vi "Setup.vi"(1 "error in":errorcluster caption="错误输入（无错误）") -> (2 "参数输出":T2={"帧ID1"=0, "等待延时"=0, "间隔延时"=0, "总时间"=0, "总次数"=0, "发送数据1"="", "接收数据1"="", "发送数据2"="", "接收数据2"="", "CAN盒类型"=3, "帧ID2"=0, "同步启动个数"=8, "模式"=enum."整体", "Baud"=12} {"Baud" items=["250k bps"=10, "10k bps"=2, "5k bps"=1, "50k bps"=5, "40k bps"=4, "20k bps"=3, "80k bps"=6, "100k bps"=7, "125k bps"=8, "200k bps"=9, "400k bps"=11, "500k bps"=12, "666k bps"=13, "800k bps"=14, "1000k bps"=15]; "帧ID2" format="%.0x"; "CAN盒类型" items=["PCI-CAN200"=7, "USB-CAN"=2, "USB-CAN200"=3]; "帧ID1" format="%.0x"}, 3 "Modify?":bool, 4 "原始参数":T2 {"CAN盒类型" items=["PCI-CAN200"=7, "USB-CAN"=2, "USB-CAN200"=3]}, 5 "error out":errorcluster caption="错误输出")   [LabVIEW 2013]
uses:
  USBCAN/DevType.ctl
panel:
  in  "输出簇":T3
  in  "Cancel":bool
  in  "Save":bool
  in  "测试参数":T2={"帧ID1"=0, "等待延时"=0, "间隔延时"=10, "总时间"=0, "总次数"=0, "发送数据1"="", "接收数据1"="", "发送数据2"="", "接收数据2"="", "CAN盒类型"=3, "帧ID2"=0, "同步启动个数"=8, "模式"=enum."整体", "Baud"=12} {"Baud" items=["250k bps"=10, "10k bps"=2, "5k bps"=1, "50k bps"=5, "40k bps"=4, "20k bps"=3, "80k bps"=6, "100k bps"=7, "125k bps"=8, "200k bps"=9, "400k bps"=11, "500k bps"=12, "666k bps"=13, "800k bps"=14, "1000k bps"=15]; "帧ID2" max=4096 step=1 format="%.0x"; "同步启动个数" min=1 max=8 step=1; "CAN盒类型" items=["PCI-CAN200"=7, "USB-CAN"=2, "USB-CAN200"=3]; "间隔延时" min=1 max=50 step=1; "帧ID1" max=4096 step=1 format="%.0x"}
  # "ms"
  # "ms"
  # "s"
  # "ms"
  # "ms"
  # "s"
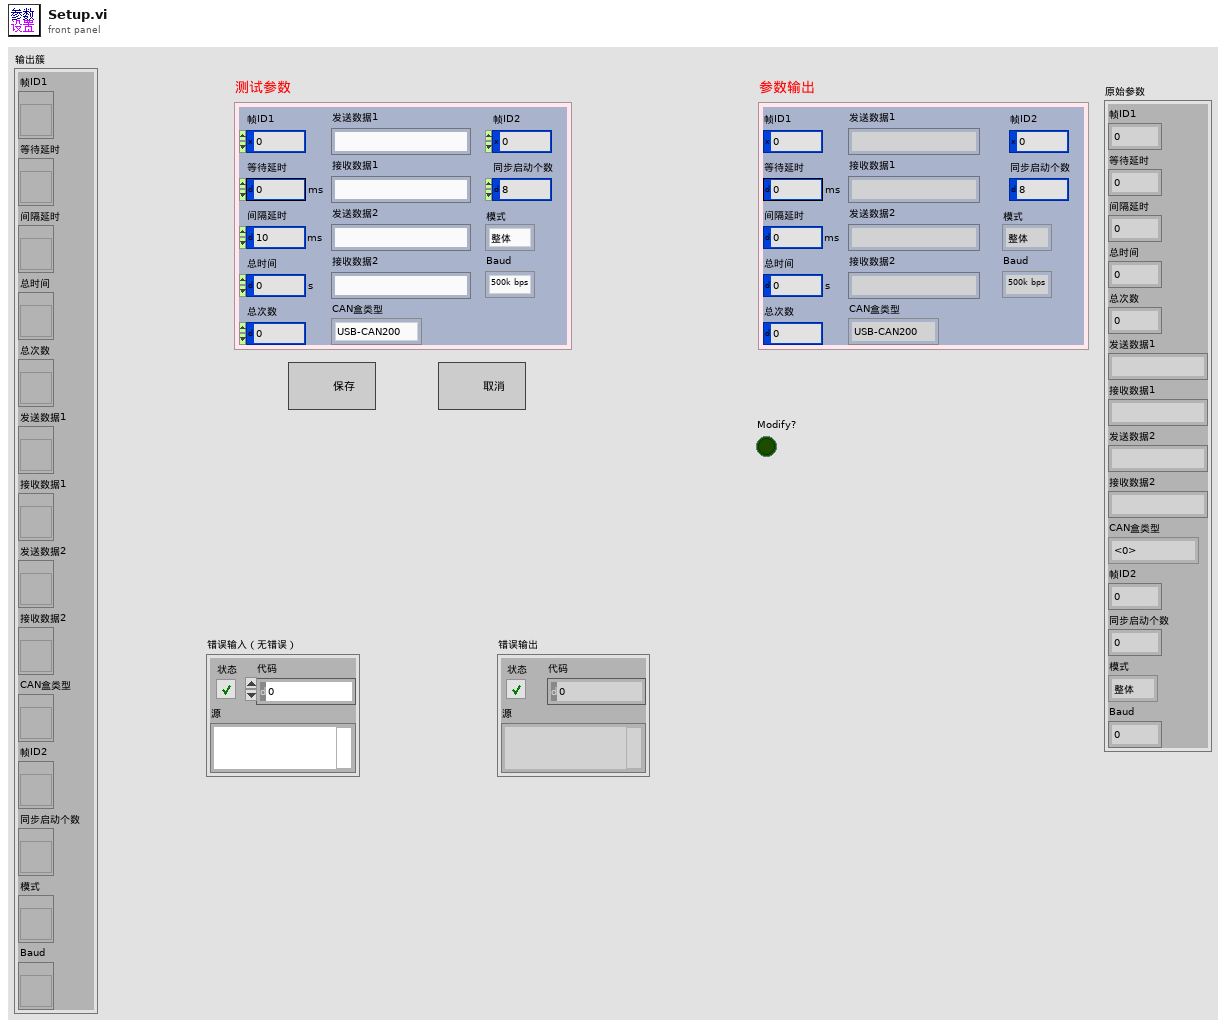
[diagram p1: front panel]
types:
  T1 = typedef "DevType.ctl" = u16
  T2 = cluster{"帧ID1":u32, "等待延时":u32, "间隔延时":u32, "总时间":u32, "总次数":u32, "发送数据1":string, "接收数据1":string, "发送数据2":string, "接收数据2":string, "CAN盒类型":T1, "帧ID2":u32, "同步启动个数":u8, "模式":enum16{"整体", "单个"}, "Baud":u8}
  T3 = cluster{"帧ID1":refnum<vi>, "等待延时":refnum<vi>, "间隔延时":refnum<vi>, "总时间":refnum<vi>, "总次数":refnum<vi>, "发送数据1":refnum<vi>, "接收数据1":refnum<vi>, "发送数据2":refnum<vi>, "接收数据2":refnum<vi>, "CAN盒类型":refnum<vi>, "帧ID2":refnum<vi>, "同步启动个数":refnum<vi>, "模式":refnum<vi>, "Baud":refnum<vi>}
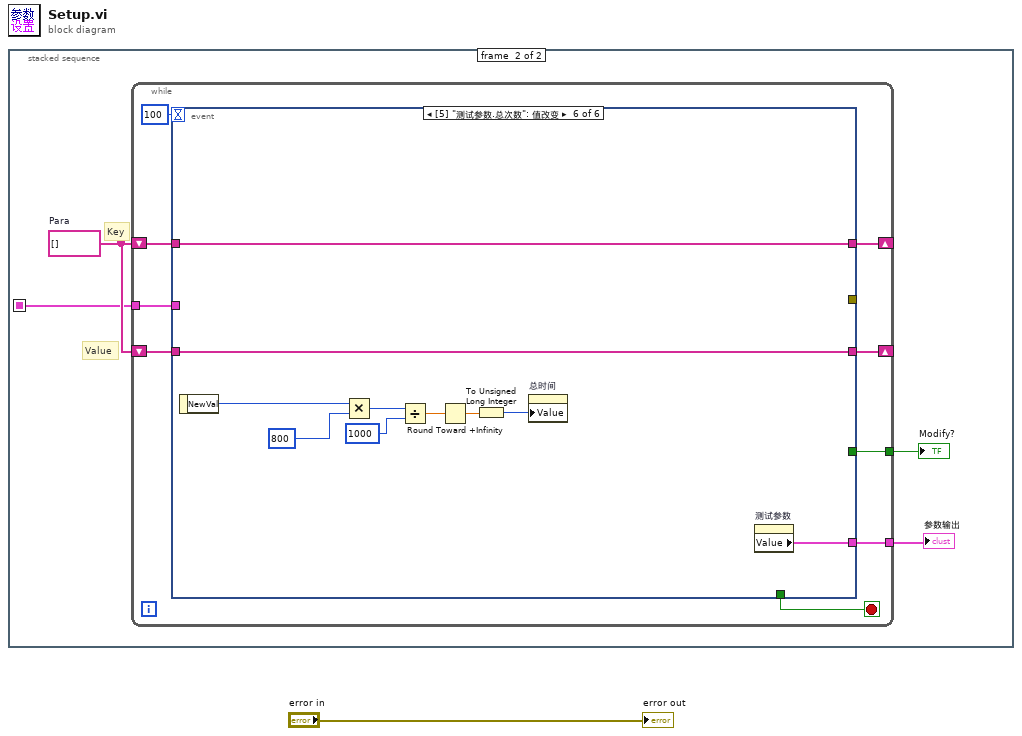
[diagram p0: block diagram]
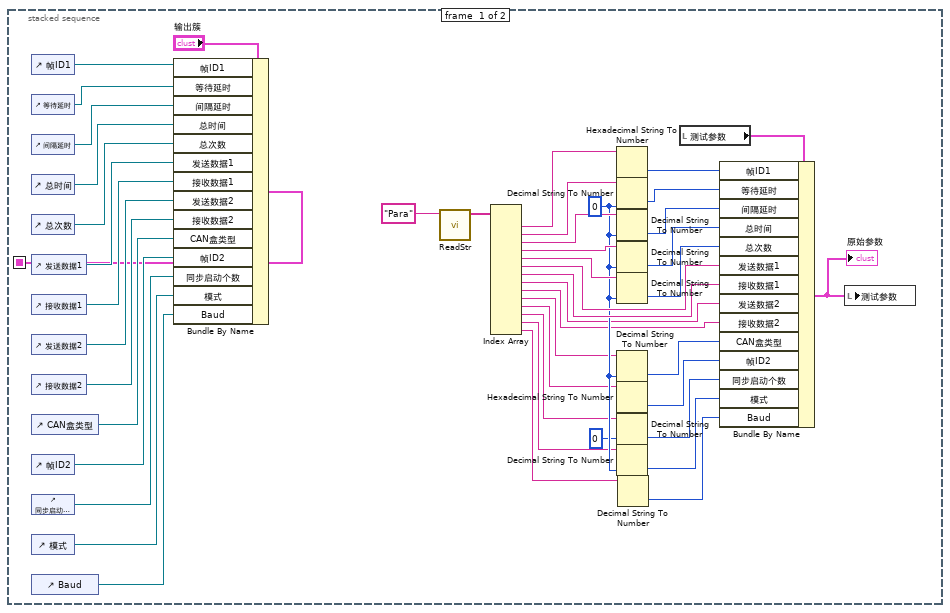
[diagram p2: hidden frame]
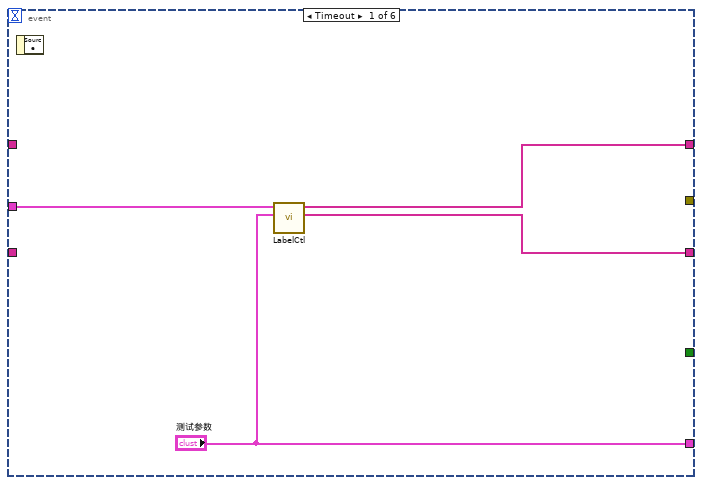
[diagram p3: hidden frame]
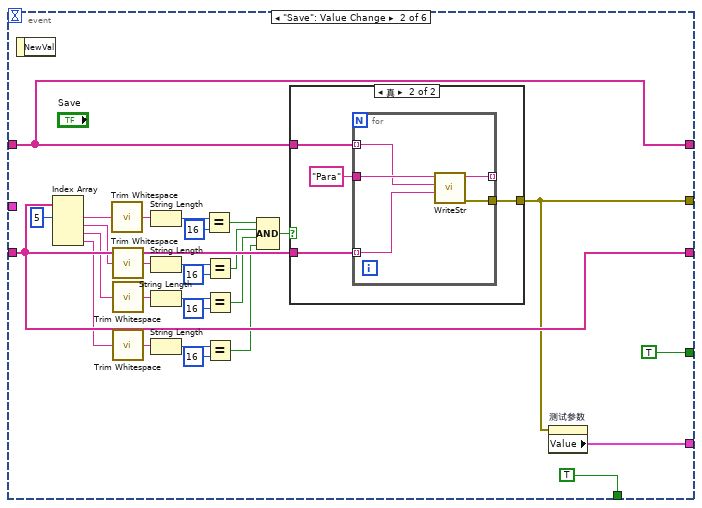
[diagram p4: hidden frame]
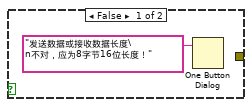
[diagram p5: hidden frame]
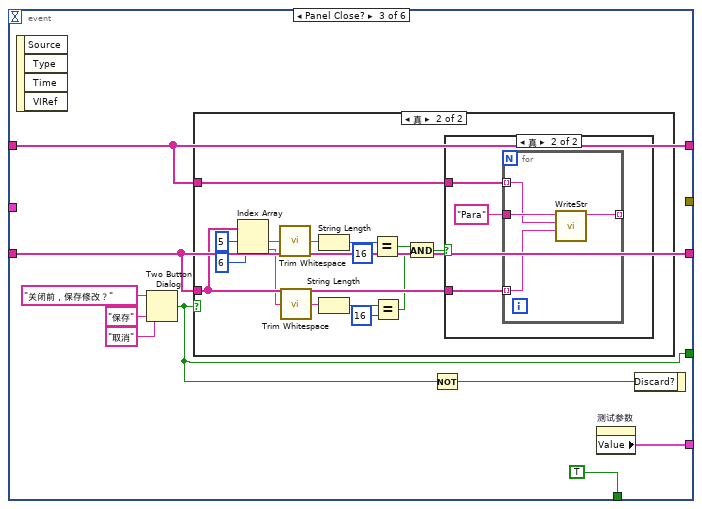
[diagram p6: hidden frame]
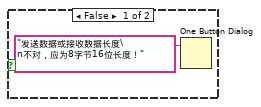
[diagram p8: hidden frame]
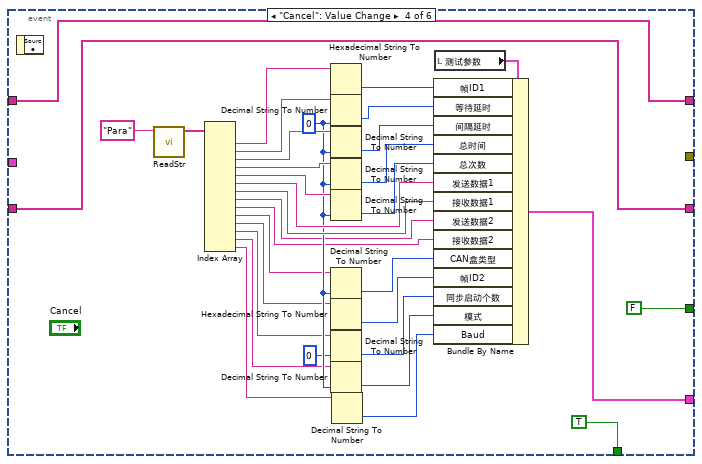
[diagram p9: hidden frame]
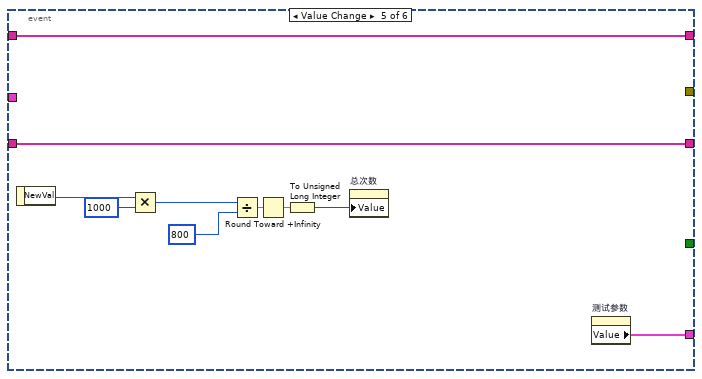
[diagram p10: hidden frame]
diagram:
  n1 = stacked-sequence {
    seq-local: [w16 _] -> [_ w49]
    frame #0 {
      w33 = u32 0
      n2 = control-ref of="帧ID1"() -> (w30:refnum<vi>)
      n3 = control-ref of="等待延时"() -> (w29:refnum<vi>)
      n4 = control-ref of="间隔延时"() -> (w28:refnum<vi>)
      n5 = control-ref of="总时间"() -> (w27:refnum<vi>)
      n6 = control-ref of="总次数"() -> (w26:refnum<vi>)
      n7 = control-ref of="发送数据1"() -> (w25:refnum<vi>)
      n8 = control-ref of="接收数据1"() -> (w24:refnum<vi>)
      n9 = control-ref of="发送数据2"() -> (w23:refnum<vi>)
      n10 = control-ref of="接收数据2"() -> (w22:refnum<vi>)
      n11 = control-ref of="CAN盒类型"() -> (w21:refnum<vi>)
      n12 = control-ref of="帧ID2"() -> (w20:refnum<vi>)
      n13 = control-ref of="同步启动个数"() -> (w19:refnum<vi>)
      n14 = control-ref of="模式"() -> (w18:refnum<vi>)
      n15 = control-ref of="Baud"() -> (w17:refnum<vi>)
      n16 = Bundle By Name(cluster="输出簇", "帧ID1"=w30, "等待延时"=w29, "间隔延时"=w28, "总时间"=w27, "总次数"=w26, "发送数据1"=w25, "接收数据1"=w24, "发送数据2"=w23, "接收数据2"=w22, "CAN盒类型"=w21, "帧ID2"=w20, "同步启动个数"=w19, "模式"=w18, "Baud"=w17) -> (w16:T3)
      n17 = call "ReadStr.vi"("section"="Para") -> ("Value"=w46:string[])  [unwired: 8 in, 2 out]
      n18 = Index Array(array=w46) -> (element #1=w45:string, element #2=w43:string, element #3=w41:string, element #4=w39:string, element #5=w37:string, element #6=w36:string, element #7=w35:string, element #8=w14:string, element #9=w13:string, element #10=w12:string, element #11=w11:string, element #12=w7:string, element #13=w6:string, element #14=w4:string)  [unwired: 14 in]
      n19 = Hexadecimal String To Number(string=w45) -> (number=w44:u32)  [unwired: 2 in, 1 out]
      n20 = Decimal String To Number(string=w43, default (0L)=w33) -> (number=w42:u32)  [unwired: 1 in, 1 out]
      n21 = Decimal String To Number(string=w41, default (0L)=w33) -> (number=w40:u32)  [unwired: 1 in, 1 out]
      n22 = Decimal String To Number(string=w39, default (0L)=w33) -> (number=w38:u32)  [unwired: 1 in, 1 out]
      n23 = Decimal String To Number(string=w37, default (0L)=w33) -> (number=w34:u32)  [unwired: 1 in, 1 out]
      n24 = Decimal String To Number(string=w12, default (0L)=w33) -> (number=w9:u32)  [unwired: 1 in, 1 out]
      n25 = Hexadecimal String To Number(string=w11) -> (number=w10:u32)  [unwired: 2 in, 1 out]
      n26 = Decimal String To Number(string=w7, default (0L)=u8 0) -> (number=w8:u8)  [unwired: 1 in, 1 out]
      n27 = Decimal String To Number(string=w6, default (0L)=w33) -> (number=w5:u32)  [unwired: 1 in, 1 out]
      n28 = Decimal String To Number(string=w4) -> (number=w3:i32)  [unwired: 2 in, 1 out]
      n29 = local read "测试参数"() -> (w15:T2)
      n30 = Bundle By Name(cluster=w15, "帧ID1"=w44, "等待延时"=w42, "间隔延时"=w40, "总时间"=w38, "总次数"=w34, "发送数据1"=w36, "接收数据1"=w35, "发送数据2"=w14, "接收数据2"=w13, "CAN盒类型"=w9, "帧ID2"=w10, "同步启动个数"=w8, "模式"=w5, "Baud"=w3) -> (w2:T2)
      "原始参数" <- w2
      n31 = local write "测试参数"(w2) -> ()
    }
    frame #1 {
      w51 = string[] []  # Para
      # "Value"
      # "Key"
      n32 = while {
        shift-right: [w60] -> _
        shift-left: w51 -> [w58]
        shift-right: [w59] -> _
        shift-left: w51 -> [w57]
        tunnel: [w54] -> w50
        tunnel: w49 -> [w53]
        tunnel: [w52] -> w48
        stop <- w56 stop-if-true
        n33 = event shown="[5] \"测试参数.总次数\": 值改变" {
          selector: _ -> [_ _ _ _ _ _]
          dyn-events: _ -> [_ _ _ _ _ _]
          timeout: 100 -> [_ _ _ _ _ _]
          tunnel: [w62 w92 w108 w168 w178 w188] -> w60
          tunnel: [w61 w91 w107 w167 w177 w187] -> w59
          tunnel: w58 -> [_ w92 w108 w168 w178 w188]
          tunnel: w57 -> [_ w91 w107 w167 w177 w187]
          tunnel: [_ TRUE TRUE TRUE _ _] -> w56
          tunnel: ["测试参数" w77 w106 w138 w176 w186] -> w54
          tunnel: w53 -> [w64 _ _ _ _ _]
          tunnel: [_ w66 _ _ _ _] -> _
          tunnel: [_ TRUE w103 FALSE _ _] -> w52
          event Timeout {
            n34 = event-data() -> ()  [unwired: 1 in, 1 out]
            n35 = call "LabelCtl.vi"("测试参数"="测试参数", "LabelIn"=w64) -> ("Value"=w61:string[], "LabelText"=w62:string[])  [unwired: 7 in, 1 out]
          }
          event "Save": Value Change {
            n36 = event-data() -> ()  [unwired: 1 in, 1 out]
            n37 = Index Array(array=w91, index #1=5 ("索引")) -> (element #1=w89:string, element #2=w88:string, element #3=w75:string, element #4=w68:string)  [unwired: 3 in]
            n38 = call <vilib>:"Trim Whitespace.vi"("string"=w89) -> ("trimmed string"=w81:string)  [unwired: 1 in]
            n39 = call <vilib>:"Trim Whitespace.vi"("string"=w88) -> ("trimmed string"=w80:string)  [unwired: 1 in]
            n40 = call <vilib>:"Trim Whitespace.vi"("string"=w75) -> ("trimmed string"=w73:string)  [unwired: 1 in]
            n41 = call <vilib>:"Trim Whitespace.vi"("string"=w68) -> ("trimmed string"=w71:string)  [unwired: 1 in]
            n42 = String Length(string=w81) -> (length=w87:i32)
            n43 = String Length(string=w80) -> (length=w86:i32)
            n44 = String Length(string=w73) -> (length=w74:i32)
            n45 = String Length(string=w71) -> (length=w70:i32)
            n46 = Equal?(x=w87, y=16 ("索引")) -> (x = y?=w84:bool)
            n47 = Equal?(x=w86, y=16 ("索引")) -> (x = y?=w82:bool)
            n48 = Equal?(x=w74, y=16 ("索引")) -> (x = y?=w72:bool)
            n49 = Equal?(x=w70, y=16 ("索引")) -> (x = y?=w67:bool)
            n50 = Compound Arithmetic op=AND(w84, w82, w72, w67) -> (w79:bool)
            n51 = case shown="真" w79 {
              tunnel: w92 -> [_ w96]
              tunnel: w91 -> [_ w95]
              tunnel: [_ w94] -> w66
              frame False {
                n52 = One Button Dialog(message="发送数据或接收数据长度\n不对，应为8字节16位长度！" ("消息")) -> ()  [unwired: 1 in, 1 out]
              }
              frame True {
                n53 = for {
                  tunnel: "Para" -> [w102]
                  tunnel: w96 -> [w101] mode=indexing
                  tunnel: w95 -> [w100] mode=indexing
                  tunnel: [w99] -> _ mode=indexing
                  tunnel: [w98] -> w94
                  n54 = call "WriteStr.vi"("value"=w100, "key"=w101, "Section"=w102) -> ("error out"=w98:errorcluster, "ConfigPath"=w99:string)  [unwired: 7 in]
                }
              }
            }
            n55 = property on="测试参数" class="Clust (严格)"(error in=w66) -> ("Value"=w77:T2)  [unwired: 1 in, 2 out]
          }
          event Panel Close? {
            n56 = event-data() -> ()  [unwired: 1 in, 4 out]
            n57 = Two Button Dialog(message="关闭前，保存修改？" ("消息"), 1:"取消" ("F按钮名称（“取消”）"), 2:"保存" ("T按钮名称（“确定”）")) -> (T button?=w103:bool)
            n58 = case shown="真" w103 {
              tunnel: w108 -> [_ w126]
              tunnel: w107 -> [_ w117]
              frame False {
              }
              frame True {
                n59 = Index Array(array=w117, index #1=5 ("索引"), index #2=6 ("索引")) -> (element #1=w124:string, element #2=w116:string)
                n60 = call <vilib>:"Trim Whitespace.vi"("string"=w124) -> ("trimmed string"=w119:string)  [unwired: 1 in]
                n61 = call <vilib>:"Trim Whitespace.vi"("string"=w116) -> ("trimmed string"=w118:string)  [unwired: 1 in]
                n62 = String Length(string=w119) -> (length=w123:i32)
                n63 = String Length(string=w118) -> (length=w122:i32)
                n64 = Equal?(x=w123, y=16 ("索引")) -> (x = y?=w114:bool)
                n65 = Equal?(x=w122, y=16 ("索引")) -> (x = y?=w113:bool)
                n66 = And(x=w114, y=w113) -> (x .and. y?=w112:bool)
                n67 = case shown="真" w112 {
                  tunnel: w126 -> [_ w130]
                  tunnel: w117 -> [_ w128]
                  frame False {
                    n68 = One Button Dialog(message="发送数据或接收数据长度\n不对，应为8字节16位长度！" ("消息")) -> ()  [unwired: 1 in, 1 out]
                  }
                  frame True {
                    n69 = for {
                      tunnel: "Para" -> [w134]
                      tunnel: w130 -> [w133] mode=indexing
                      tunnel: w128 -> [w132] mode=indexing
                      tunnel: [w131] -> _ mode=indexing
                      n70 = call "WriteStr.vi"("value"=w132, "key"=w133, "Section"=w134) -> ("ConfigPath"=w131:string)  [unwired: 7 in, 1 out]
                    }
                  }
                }
              }
            }
            n71 = Not(x=w103) -> (.not. x?=w105:bool)
            n72 = property on="测试参数" class="Clust (严格)"() -> ("Value"=w106:T2)  [unwired: 2 in, 2 out]
            n73 = event-data("Discard?"=w105) -> ()  [unwired: 1 in, 1 out]
          }
          event "Cancel": Value Change {
            w153 = u32 0
            n74 = event-data() -> ()  [unwired: 1 in, 1 out]
            n75 = call "ReadStr.vi"("section"="Para") -> ("Value"=w164:string[])  [unwired: 8 in, 2 out]
            n76 = Index Array(array=w164) -> (element #1=w139:string, element #2=w163:string, element #3=w161:string, element #4=w159:string, element #5=w157:string, element #6=w156:string, element #7=w155:string, element #8=w151:string, element #9=w150:string, element #10=w149:string, element #11=w148:string, element #12=w144:string, element #13=w143:string, element #14=w141:string)  [unwired: 14 in]
            n77 = Hexadecimal String To Number(string=w139) -> (number=w136:u32)  [unwired: 2 in, 1 out]
            n78 = Decimal String To Number(string=w163, default (0L)=w153) -> (number=w162:u32)  [unwired: 1 in, 1 out]
            n79 = Decimal String To Number(string=w161, default (0L)=w153) -> (number=w160:u32)  [unwired: 1 in, 1 out]
            n80 = Decimal String To Number(string=w159, default (0L)=w153) -> (number=w158:u32)  [unwired: 1 in, 1 out]
            n81 = Decimal String To Number(string=w157, default (0L)=w153) -> (number=w154:u32)  [unwired: 1 in, 1 out]
            n82 = Decimal String To Number(string=w149, default (0L)=w153) -> (number=w146:u32)  [unwired: 1 in, 1 out]
            n83 = Hexadecimal String To Number(string=w148) -> (number=w147:u32)  [unwired: 2 in, 1 out]
            n84 = Decimal String To Number(string=w144, default (0L)=u8 0) -> (number=w145:u8)  [unwired: 1 in, 1 out]
            n85 = Decimal String To Number(string=w143, default (0L)=w153) -> (number=w142:u32)  [unwired: 1 in, 1 out]
            n86 = Decimal String To Number(string=w141) -> (number=w140:i32)  [unwired: 2 in, 1 out]
            n87 = local read "测试参数"() -> (w137:T2)
            n88 = Bundle By Name(cluster=w137, "帧ID1"=w136, "等待延时"=w162, "间隔延时"=w160, "总时间"=w158, "总次数"=w154, "发送数据1"=w156, "接收数据1"=w155, "发送数据2"=w151, "接收数据2"=w150, "CAN盒类型"=w146, "帧ID2"=w147, "同步启动个数"=w145, "模式"=w142, "Baud"=w140) -> (w138:T2)
          }
          event "测试参数.总时间": Value Change {
            n89 = event-data() -> ("NewVal"=w175:u32)  [unwired: 1 in]
            n90 = Multiply(x=w175, y=u32 1000) -> (x*y=w173:u32)
            n91 = Divide(x=w173, y=u32 800) -> (x/y=w171:dbl)
            n92 = Round Toward +Infinity(x=w171) -> (ceil(x): smallest int >= x=w170:dbl)
            n93 = To Unsigned Long Integer(number=w170) -> (unsigned 32bit integer=w172:u32)
            n94 = property on="总次数" class="DigNum (严格)"("Value"=w172) -> ()  [unwired: 2 in, 2 out]
            n95 = property on="测试参数" class="Clust (严格)"() -> ("Value"=w176:T2)  [unwired: 2 in, 2 out]
          }
          event "测试参数.总次数": Value Change {
            n96 = event-data() -> ("NewVal"=w185:u32)  [unwired: 1 in]
            n97 = Multiply(x=w185, y=800) -> (x*y=w184:u32)
            n98 = Divide(x=w184, y=1000) -> (x/y=w182:dbl)
            n99 = Round Toward +Infinity(x=w182) -> (ceil(x): smallest int >= x=w181:dbl)
            n100 = To Unsigned Long Integer(number=w181) -> (unsigned 32bit integer=w180:u32)
            n101 = property on="总时间" class="DigNum (严格)"("Value"=w180) -> ()  [unwired: 2 in, 2 out]
            n102 = property on="测试参数" class="Clust (严格)"() -> ("Value"=w186:T2)  [unwired: 2 in, 2 out]
          }
        }
      }
      "参数输出" <- w50
      "Modify?" <- w48
    }
  }
  "error out" <- "error in"
